vi "Send.vi"(7 "Message Priority (Normal)":T1=enum."Normal", 8 "error in (no error)":errorcluster, 9 "Message":refnum<class "Message.lvclass">, 10 "Actor in":refnum<class "Actor.lvclass">, 11 "Addressed Msg in":refnum<class "Addressed Msg.lvclass">) -> (0 "error out":errorcluster, 1 "Dropped?":bool, 2 "Actor out":refnum<class "Actor.lvclass">)   [LabVIEW 2020, in "Publisher.lvlib" / "Addressed Msg.lvclass"]
doc: "Send a Message somewhere through the Publisher. \n\nThis implementation sends an Addressed Msg if the Enqeuer ID string is not empty."
uses:
  Addressed Msg.lvclass
  C:/Current projects/WS/Framework/Framework/Actors/Publisher/Publisher Messages/Sender Msg/Sender Msg.lvclass
  C:/Current projects/WS/Framework/Framework/Actors/Publisher/Publisher Messages/Publisher Msg/Publisher Msg.lvclass
  PPL/HDH.Actor Framework.Core.Actor.lvlibp/1abvi3w/vi.lib/ActorFramework/Message Enqueuer/Message Priority.ctl
  PPL/HDH.Actor Framework.Core.Actor.lvlibp/1abvi3w/vi.lib/ActorFramework/Message/Message.lvclass
  PPL/HDH.Actor Framework.Core.Actor.lvlibp/1abvi3w/vi.lib/ActorFramework/Actor/Actor.lvclass
  Addressed Msg.lvclass/Addressed Msg.ctl
  Sender Msg/Sender Msg.lvclass/Sender Msg.ctl
  Publisher Msg/Publisher Msg.lvclass
  Sender Msg/Sender Msg.lvclass
  PPL/HDH.Actor Framework.Core.Actor.lvlibp/1abvi3w/vi.lib/ActorFramework/Message Enqueuer/Message Enqueuer.lvclass
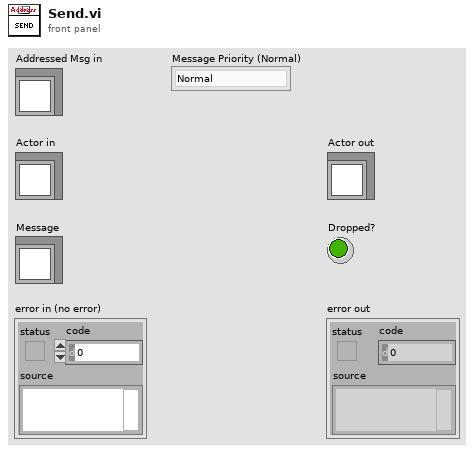
[diagram p1: front panel]
types:
  T1 = typedef "HDH.Actor Framework.Core.Actor.lvlibp/Message Enqueuer.lvclass/Message Priority.ctl" = enum16{"Low", "Normal", "High"}
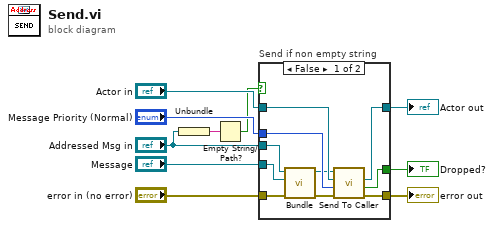
[diagram p0: block diagram]
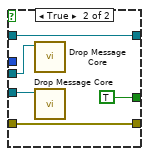
[diagram p2: hidden frame]
diagram:
  n1 = Unbundle("Addressed Msg in") -> (w2:string)
  n2 = Empty String/Path?(string/path=w2) -> (empty?=w1:bool)
  n3 = case "Send if non empty string" shown="False" w1 {
    tunnel: "Message Priority (Normal)" -> [w20 _]
    tunnel: "Actor in" -> [w19 w25]
    tunnel: [w18 w25] -> w9
    tunnel: "Message" -> [w17 w23]
    tunnel: "error in (no error)" -> [w16 w21]
    tunnel: [w13 TRUE ("Msg Dropped?")] -> w8
    tunnel: [w12 w21] -> w4
    tunnel: "Addressed Msg in" -> [w11 w24]
    frame False {
      n4 = call "Bundle.vi"("error in (no error)"=w16, "Message"=w17, "Targetted Msg in"=w11) -> ("error out"=w14:errorcluster, "Targetted Msg out"=w15:refnum<class "Addressed Msg.lvclass">)  [unwired: 7 in]
      n5 = call "Send To Caller.vi"("error in (no error)"=w14, "Message Priority (Normal)"=w20, "Actor in"=w19, "Publisher Msg in"=w15) -> ("error out"=w12:errorcluster, "Msg Dropped?"=w13:bool, "Actor out"=w18:refnum<class "Actor.lvclass">)  [unwired: 5 in]
    }
    frame True {
      n6 = call-dynamic "Drop Message Core.vi"("Message in"=w24) -> ()  [unwired: 11 in]
      n7 = call-dynamic "Drop Message Core.vi"("Message in"=w23) -> ()  [unwired: 11 in]
    }
  }
  "error out" <- w4
  "Actor out" <- w9
  "Dropped?" <- w8
